vi "Queue_Send_Data.vi"(8 "错误输入（无错误）":errorcluster, 11 "Communication message":T1) -> (0 "错误输出":errorcluster)   [LabVIEW 2014]
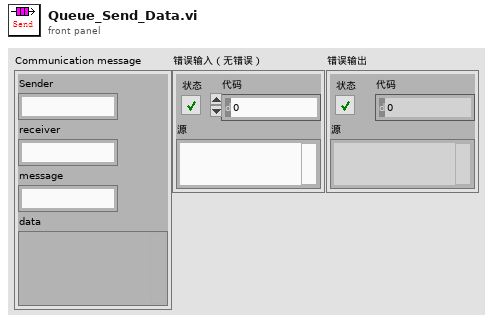
[diagram p1: front panel]
types:
  T1 = cluster{"Sender":string, "receiver":string, "message":string, "data":variant}
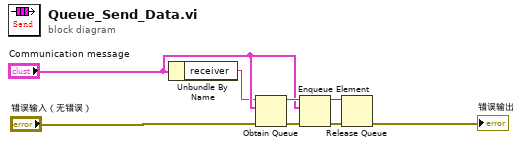
[diagram p0: block diagram]
diagram:
  n1 = Unbundle By Name("Communication message") -> ("receiver"=w1:string)
  n2 = Obtain Queue(name (unnamed)=w1, element data type="Communication message", error in (no error)="错误输入（无错误）") -> (queue out=w5:refnum<queue>, error out=w6:errorcluster)  [unwired: 2 in, 1 out]
  n3 = Enqueue Element(queue=w5, element="Communication message", error in (no error)=w6) -> (queue out=w7:refnum<queue>, error out=w8:errorcluster)  [unwired: 1 in, 1 out]
  n4 = Release Queue(queue=w7, error in (no error)=w8) -> (error out=→"错误输出":errorcluster)  [unwired: 1 in, 2 out]
